vi "run_experiment_multi_mix_v2.vi"(4 "Sync Camera Acquisition":bool, 5 "Video File Name":path, 7 "Pressure Sequence":dbl[][](array[numeric]), 8 "Valve Sequence Data":T2(array[cluster]), 9 "mixture sequence array":string[](array[string]), 10 "Time Sequence":dbl[](array[numeric]), 11 "MFCS_EZ":T3) -> (0 "Aborted?":bool, 3 "Flow Data Out":T1)   [LabVIEW 2016]
uses:
  <userlib>/Fluigent/Fluigent MFCS/FluigentMFCS_Full.llb/_EZmfcsRefNum.ctl
  <userlib>/Fluigent/Fluigent MFCS/FluigentMFCS_Full.llb/_EZmfcsEnum.ctl
  <userlib>/Fluigent/Fluigent MFCS/FluigentMFCS_Full.llb/MFCS_EZ Write Channel Pressure.vi
  Globals/PressuresGlobal.vi
panel:
  out "Previous state":string
  out "Next State":string
  out "x-y":u32
  out "Video File Name":path
  in  "stop":bool
  out "Step Time":u8(slide) scale=0.0..100.0
  out "Current State":string
  out "Remaining Time":dbl
  out "Experiment Progress":u8(slide) scale=0.0..100.0
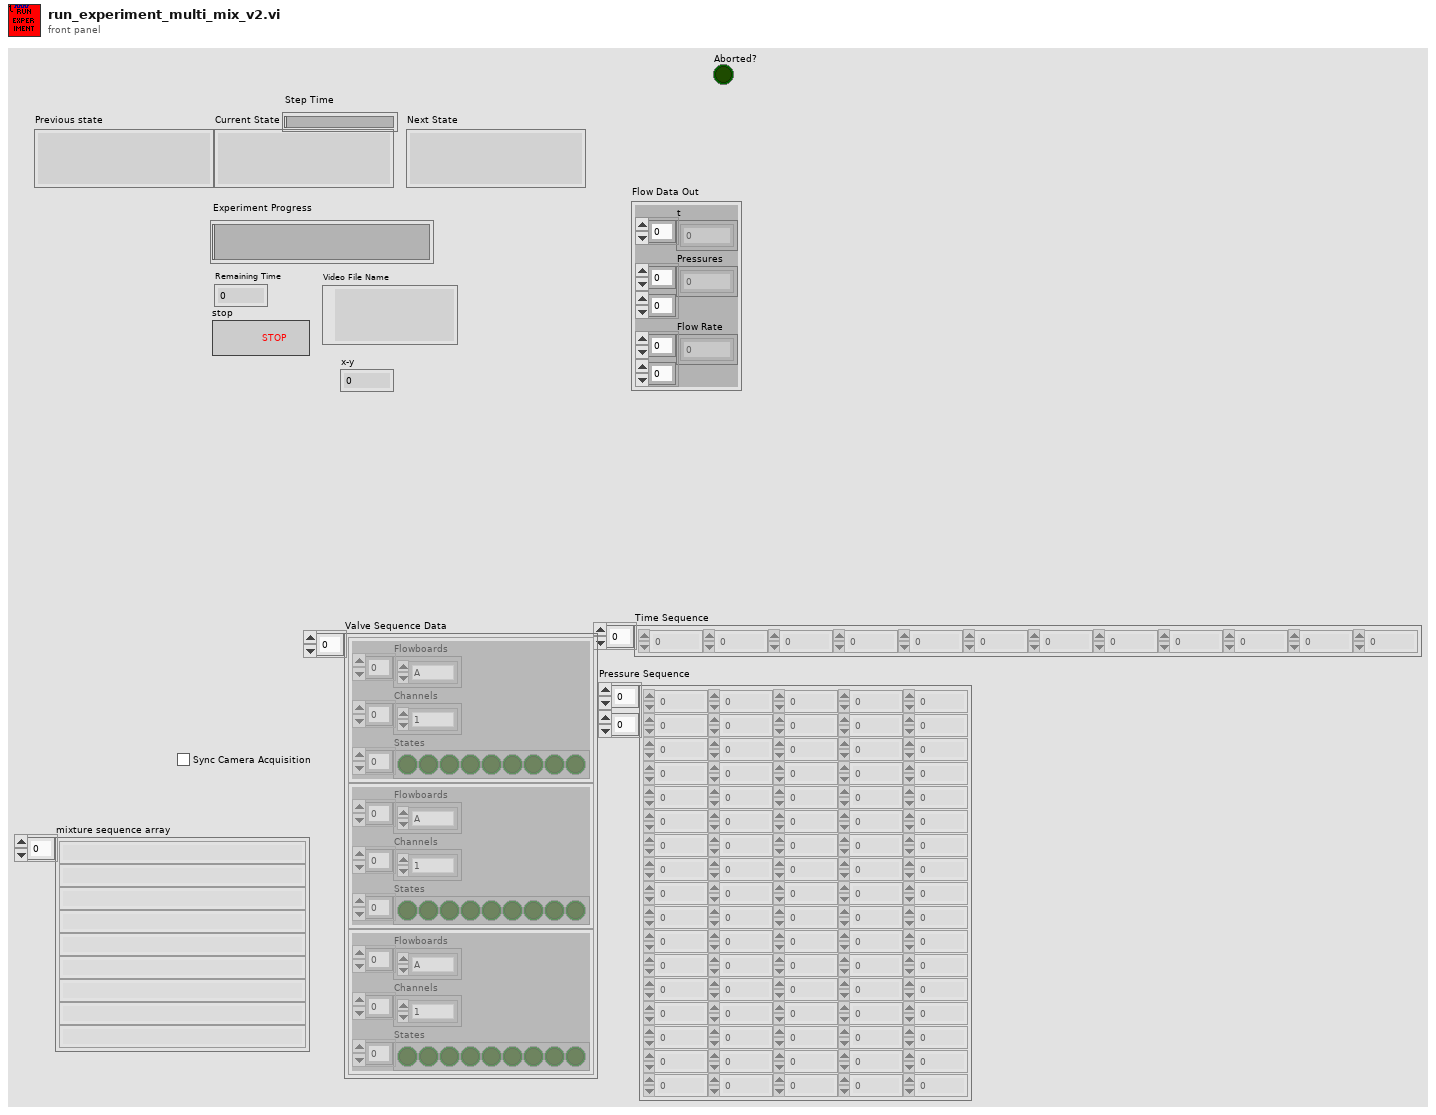
[diagram p1: front panel]
types:
  T1 = cluster{"t":dbl[], "Pressures":dbl[][], "Flow Rate":dbl[][]}
  T2 = cluster{"Flowboards":enum16{"A", "B", "C"}[], "Channels":enum16{"1", "2", "3", "4", "5", "6", "7", "8"}[], "States":bool[]}[]
  T3 = typedef "_EZmfcsRefNum.ctl" = refnum<k1>
  T4 = enum16{"Release", "Create", "Send", "Wait", "Cancel"}
  T5 = cluster{"Flowboards":enum16{"A", "B", "C"}[], "Channels":enum16{"1", "2", "3", "4", "5", "6", "7", "8"}[], "States":bool[]}
  T6 = cluster{"Video File Name":path, "Start Water":dbl}
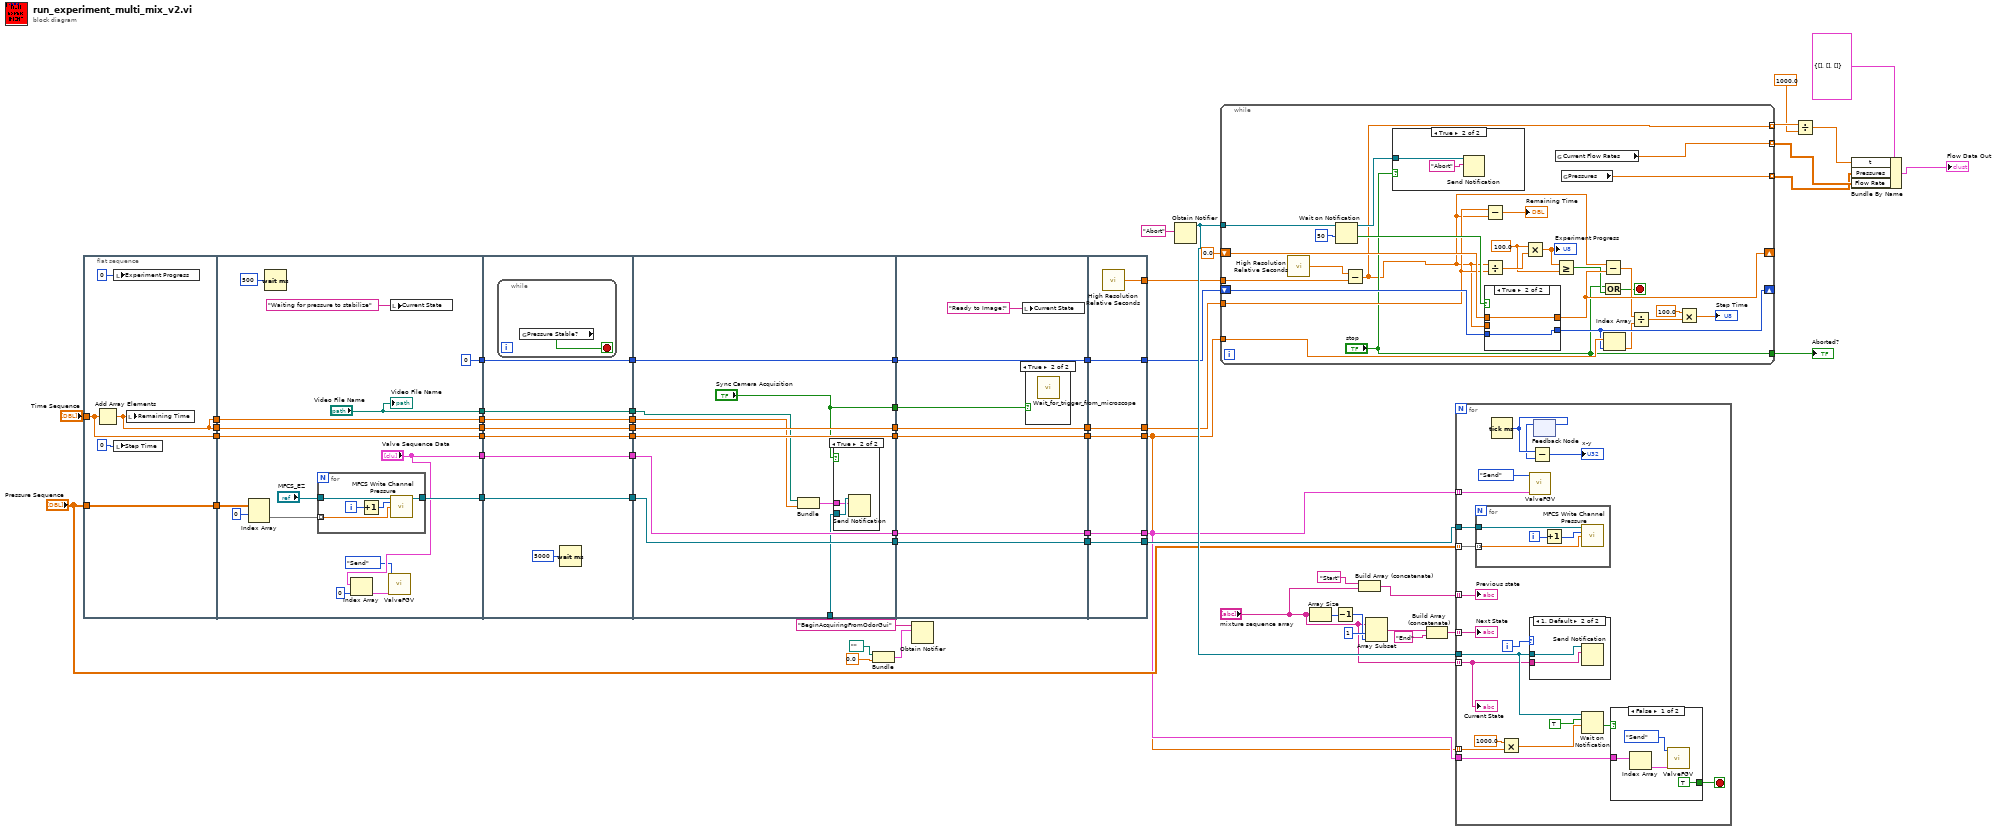
[diagram p0: block diagram]
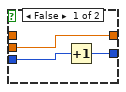
[diagram p5: hidden frame]
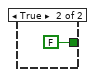
[diagram p7: hidden frame]
diagram:
  n1 = flat-sequence {
    tunnel: "Pressure Sequence" -> [w67]
    tunnel: [w67] -> w58
    tunnel: "Time Sequence" -> [w64]
    tunnel: [w64] -> w53
    tunnel: [w63] -> w52
    tunnel: [w63] -> w33
    tunnel: w58 -> [w74]
    tunnel: [w80] -> w50
    tunnel: ["Valve Sequence Data"] -> w49
    tunnel: [0] -> w48
    tunnel: [w78] -> w47
    tunnel: [w77] -> w46
    tunnel: w53 -> [w78]
    tunnel: w52 -> [w77]
    tunnel: [w76] -> w34
    tunnel: w33 -> [w76]
    tunnel: ["Video File Name"] -> w20
    tunnel: w50 -> [w96]
    tunnel: [w96] -> w41
    tunnel: w49 -> [w95]
    tunnel: [w95] -> w40
    tunnel: w48 -> [w94]
    tunnel: [w94] -> w39
    tunnel: w47 -> [w93]
    tunnel: [w93] -> w38
    tunnel: w46 -> [w92]
    tunnel: [w92] -> w37
    tunnel: [w91] -> w35
    tunnel: w34 -> [w91]
    tunnel: [w90] -> w21
    tunnel: w20 -> [w90]
    tunnel: w41 -> [w107]
    tunnel: [w107] -> w32
    tunnel: w40 -> [w106]
    tunnel: [w106] -> w30
    tunnel: w39 -> [w105]
    tunnel: [w105] -> w28
    tunnel: w38 -> [w104]
    tunnel: [w104] -> w26
    tunnel: w37 -> [w103]
    tunnel: [w103] -> w24
    tunnel: w36 -> [w101]
    tunnel: w35 -> [w100]
    tunnel: ["Sync Camera Acquisition"] -> w22
    tunnel: w21 -> [w98]
    tunnel: w32 -> [w116]
    tunnel: [w116] -> w31
    tunnel: w30 -> [w115]
    tunnel: [w115] -> w29
    tunnel: w28 -> [w114]
    tunnel: [w114] -> w27
    tunnel: w26 -> [w113]
    tunnel: [w113] -> w25
    tunnel: w24 -> [w112]
    tunnel: [w112] -> w23
    tunnel: w22 -> [w111]
    tunnel: [w118] -> w56
    tunnel: [w119] -> w11
    tunnel: [w120] -> w57
    tunnel: [w121] -> w12
    tunnel: [w122] -> w59
    tunnel: w31 -> [w122]
    tunnel: w29 -> [w121]
    tunnel: w27 -> [w120]
    tunnel: w25 -> [w119]
    tunnel: w23 -> [w118]
    tunnel: [w117] -> w55
    frame #0 {
      n2 = Add Array Elements(numeric array=w64) -> (sum=w63:dbl)
      n3 = local write "Experiment Progress"(u8 0 ("Experiment Progress")) -> ()
      n4 = local write "Step Time"(u8 0 ("Step Time")) -> ()
      n5 = local write "Remaining Time"(w63) -> ()
    }
    frame #1 {
      n6 = Index Array(array=w74, index (row)=0) -> (element=w72:dbl[])  [unwired: 1 in]
      n7 = Wait (ms)(milliseconds to wait=u32 500) -> ()  [unwired: 1 out]
      n8 = for {
        tunnel: "MFCS_EZ" -> [w88]
        tunnel: w72 -> [w87] mode=indexing
        tunnel: [w86] -> w80
        i -> [w85]
        n9 = Increment(x=w85) -> (x+1=w84:i32)
        n10 = call-poly <userlib>:"MFCS Write Channel Pressure.vi"("MFCS_EZ"=w88, "Channel Number (default=1)"=w84, "Pressure (mBar)"=w87) -> ("MFCS_EZ out"=w86:T3)  [unwired: 11 in, 1 out]
      }
      n11 = Index Array(array="Valve Sequence Data", index=0) -> (element=w71:T5)
      n12 = call "ValveFGV.vi"("Valve Data"=w71, "Action"=T4."Send") -> ()  [unwired: 6 in, 4 out]
      n13 = local write "Current State"("Waiting for pressure to stabilize" ("Current State")) -> ()
      "Video File Name" <- "Video File Name"
    }
    frame #2 {
      n14 = while {
        stop <- w97 stop-if-true
        n15 = global read "PressuresGlobal.vi" "Pressure Stable?"() -> (w97:bool)
      }
      n16 = Wait (ms)(milliseconds to wait=u32 5000) -> ()  [unwired: 1 out]
    }
    frame #3 {
      n17 = Bundle("Video File Name"=w98, "Start Water"=w100) -> (w102:T6)  [unwired: 1 in]
      n18 = case shown="True" "Sync Camera Acquisition" {
        tunnel: w101 -> [_ w109]
        tunnel: w102 -> [_ w108]
        frame False {
        }
        frame True {
          n19 = Send Notification(notification=w108, notifier=w109) -> ()  [unwired: 1 in, 2 out]
        }
      }
    }
    frame #4 {
      n20 = local write "Current State"("Ready to Image!" ("Current State")) -> ()
      n21 = case shown="True" w111 {
        frame False {
        }
        frame True {
          n22 = call "Wait_for_trigger_from_microscope.vi"() -> ()  [unwired: 12 in]
        }
      }
    }
    frame #5 {
      n23 = call <vilib>:"High Resolution Relative Seconds.vi"() -> ("relative seconds"=w117:dbl)
    }
  }
  n24 = Bundle("Log File Name"=path "", 0.0) -> (w43:cluster{"Log File Name":path, dbl})  [unwired: 1 in]
  n25 = Obtain Notifier(name (unnamed)="BeginAcquiringFromOdorGui", notification data type=w43) -> (notifier out=w36:refnum<notifier>)  [unwired: 2 in, 2 out]
  n26 = Obtain Notifier(notification data type="Abort" ("notification")) -> (notifier out=w62:refnum<notifier>)  [unwired: 3 in, 2 out]
  n27 = while {
    tunnel: w62 -> [w146]
    tunnel: w56 -> [w137]
    tunnel: w55 -> [w149]
    tunnel: w11 -> [w142]
    shift-right: [w133] -> _
    shift-left: 0.0 -> [w143]
    shift-right: [w140] -> _
    shift-left: w57 -> [w141]
    tunnel: ["stop"] -> w51
    tunnel: [w126] -> w15 mode=indexing
    tunnel: [w123] -> w19 mode=indexing
    tunnel: [w124] -> w14 mode=indexing
    stop <- w128 stop-if-true
    w130 = 100.0 ("x")
    n28 = call <vilib>:"High Resolution Relative Seconds.vi"() -> ("relative seconds"=w125:dbl)
    n29 = Wait on Notification(notifier=w146, timeout in ms (-1)=50) -> (notifier out=w138:refnum<notifier>, timed out?=w144:bool)  [unwired: 2 in, 2 out]
    n30 = Subtract(x=w125, y=w149) -> (x-y=w123:dbl)
    n31 = case shown="True" "stop" {
      tunnel: w138 -> [_ w151]
      frame False {
      }
      frame True {
        n32 = Send Notification(notification="Abort", notifier=w151) -> ()  [unwired: 1 in, 2 out]
      }
    }
    n33 = Subtract(x=w137, y=w123) -> (x-y=→"Remaining Time":dbl)
    n34 = Divide(x=w123, y=w137) -> (x/y=w147:dbl)
    n35 = case shown="True" w144 {
      tunnel: w123 -> [w154 _]
      tunnel: [w154 w156] -> w133
      tunnel: w143 -> [_ w156]
      tunnel: w141 -> [w153 w155]
      tunnel: [w152 w155] -> w140
      frame False {
        n36 = Increment(x=w153) -> (x+1=w152:i32)
      }
      frame True {
      }
    }
    n37 = Multiply(x=w130, y=w147) -> (x*y=w131:dbl)
    "Experiment Progress" <- w131
    n38 = Greater Or Equal?(x=w131, y=w130) -> (x >= y?=w129:bool)
    n39 = global read "PressuresGlobal.vi" "Current Flow Rates"() -> (w126:dbl[])
    n40 = global read "PressuresGlobal.vi" "Pressures"() -> (w124:dbl[])
    n41 = Subtract(x=w123, y=w133) -> (x-y=w132:dbl)
    n42 = Or(x="stop", y=w129) -> (x .or. y?=w128:bool)
    n43 = Index Array(array=w142, index=w140) -> (element=w139:dbl)
    n44 = Divide(x=w132, y=w139) -> (x/y=w135:dbl)
    n45 = Multiply(x=100.0, y=w135) -> (x*y=→"Step Time":dbl)
  }
  "Aborted?" <- w51
  n46 = Array Size(array="mixture sequence array") -> (size(s)=w8:i32)
  n47 = Decrement(x=w8) -> (x-1=w7:i32)
  n48 = Build Array (concatenate)("Start", "mixture sequence array") -> (w3:string[])
  n49 = Array Subset(array="mixture sequence array", index=1, length=w7) -> (w5:string[])
  n50 = Build Array (concatenate)(w5, "End") -> (w4:string[])
  n51 = for {
    tunnel: w62 -> [w167]
    tunnel: w11 -> [w159] mode=indexing
    tunnel: w12 -> [w164] mode=indexing
    tunnel: "mixture sequence array" -> [w166] mode=indexing
    tunnel: "Pressure Sequence" -> [w169] mode=indexing
    tunnel: w59 -> [w168]
    tunnel: w12 -> [w163]
    tunnel: w3 -> [w158] mode=indexing
    tunnel: w4 -> [w157] mode=indexing
    i -> [w165]
    stop <- w174 stop-if-true
    n52 = for {
      tunnel: w168 -> [w181]
      tunnel: w169 -> [w180] mode=indexing
      i -> [w179]
      n53 = Increment(x=w179) -> (x+1=w178:i32)
      n54 = call-poly <userlib>:"MFCS Write Channel Pressure.vi"("MFCS_EZ"=w181, "Channel Number (default=1)"=w178, "Pressure (mBar)"=w180) -> ()  [unwired: 11 in, 2 out]
    }
    n55 = Tick Count (ms)() -> (millisecond timer value=w173:u32)
    n56 = Multiply(x=1000.0, y=w159) -> (x*y=w162:dbl)
    n57 = call "ValveFGV.vi"("Valve Data"=w164, "Action"=T4."Send") -> ()  [unwired: 6 in, 4 out]
    n58 = case shown="1, Default" w165 {
      tunnel: w167 -> [_ w177]
      tunnel: w166 -> [_ w176]
      frame 0 {
      }
      frame 1, Default {
        n59 = Send Notification(notification=w176, notifier=w177) -> ()  [unwired: 1 in, 2 out]
      }
    }
    n60 = feedback #1() -> (w172:u32)  [unwired: 1 in]
    n61 = Subtract(x=w173, y=w172) -> (x-y=→"x-y":u32)
    n62 = feedback-in #1(w173) -> ()
    n63 = Wait on Notification(notifier=w167, ignore previous (F)=TRUE, timeout in ms (-1)=w162) -> (timed out?=w175:bool)  [unwired: 1 in, 3 out]
    n64 = case shown="False" w175 {
      tunnel: [TRUE FALSE] -> w174
      tunnel: w163 -> [w183 _]
      frame False {
        n65 = Index Array(array=w183) -> (element=w182:T5)  [unwired: 1 in]
        n66 = call "ValveFGV.vi"("Valve Data"=w182, "Action"=T4."Send") -> ()  [unwired: 6 in, 4 out]
      }
      frame True {
      }
    }
    "Current State" <- w166
    "Next State" <- w157
    "Previous state" <- w158
  }
  n67 = Divide(x=w19, y=1000.0) -> (x/y=w16:dbl[])
  n68 = Bundle By Name(cluster=T1 {"t"=[], "Pressures"=[], "Flow Rate"=[]} ("Flow Data Out"), "t"=w16, "Pressures"=w14, "Flow Rate"=w15) -> (→"Flow Data Out":T1)
